vi "单参数加标流程.vi"(10 "流程类型":T1(ring), 11 "Slave ID":T3=enum."氨氮") -> ()   [LabVIEW 2016, in "质控单元V4.lvlib"]
panel:
  out "加标回收启动时间":timestamp
  out "水样测试启动时间":timestamp
  out "Next State":string
  in  "仪器加标回收启动计数":u16
  in  "仪器水样测试启动计数":u16
  in  "加标模块排液启动计数":u16
  in  "加标模块加标启动计数":u16
  in  "加标模块进样启动计数":u16
  in  "加标模块润洗启动计数":u16
  in  "采配水启动次数计数":u16
  in  "加标回收测试时间":timestamp
  in  "水样测试时间":timestamp
  in  "质控数据":T2
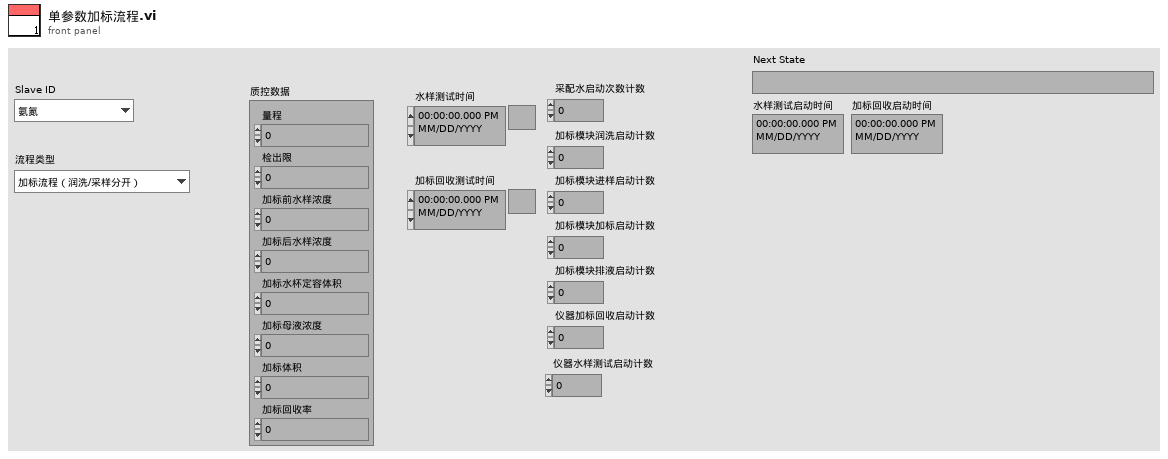
[diagram p1: front panel]
types:
  T1 = enum16{"加标流程（润洗/采样分开）", "加标流程（润洗/采样合并）", "加标流程（不启动采配水）", "水样测试（润洗/采样分开）", "水样测试（润洗/采样合并）", "水样测试（不启动采配水）"}
  T2 = cluster{"量程":dbl, "检出限":dbl, "加标前水样浓度":dbl, "加标后水样浓度":dbl, "加标水杯定容体积":dbl, "加标母液浓度":dbl, "加标体积":dbl, "加标回收率":dbl}
  T3 = typedef "质控单元V4.lvlib/质控slave id.ctl" = enum16{"null", "氨氮", "总磷", "总氮", "CODMn", "CODCr", "氨氮总磷", "总磷总氮"}
  T4 = cluster{"氨氮":bool, "总磷":bool, "总氮":bool, "CODMn":bool, "CODCr":bool, "氨氮总磷":bool, "总磷总氮":bool}
  T5 = cluster{"时间":timestamp, "参数":string, "数据类型":string, "加标前水样测试时间":timestamp, "加标前水样浓度值":sgl, "加标后水样浓度值":sgl, "加标母液浓度值":sgl, "加标体积":sgl, "加标水杯定容体积":sgl, "加标回收率":sgl}
  T6 = enum16{"待机", "润洗", "采样", "沉淀", "配水", "反冲洗", "储水", "结束"}
  T7 = typedef "质控单元V4.lvlib/质控流程控制.ctl" = enum16{"待机", "启动进样流程", "启动加标流程", "启动排液流程", "启动润洗流程", "停止流程"}
  T8 = enum16{"待机", "润洗", "进样", "定量", "加标", "等待取样", "排液", "异常停机"}
  T9 = enum16{"空闲", "水样测试", "标样核查", "零点核查", "跨度核查", "空白测试", "平行样测试", "加标回收", "空白校准", "标样校准", "初始化（清洗）"}
  T10 = cluster{"水样数据时间":timestamp, "水样实测值":sgl, "水样数据标识":string}
  T11 = cluster{"加标回收数据时间":timestamp, "加标回收实测值":sgl, "加标回收数据标识":string}
  T12 = typedef "质控单元V4.lvlib/质控仪器状态.ctl" = cluster{"运行状态":enum16{"待机", "润洗", "进样", "定量", "加标", "等待取样", "排液", "异常停机"}, "液位状态":enum16{"无感应", "有感应"}, "告警状态":enum16{"无告警", "液位故障告警", "注射泵异常"}, "当前步骤数":u16, "当前步骤剩余时间":u16, "当前步骤具体操作":enum16{"加标", "进样", "排液", "搅拌", "定量"}, "当前流程":enum16{"待机", "进样流程", "加标流程", "排液流程", "润洗流程"}}
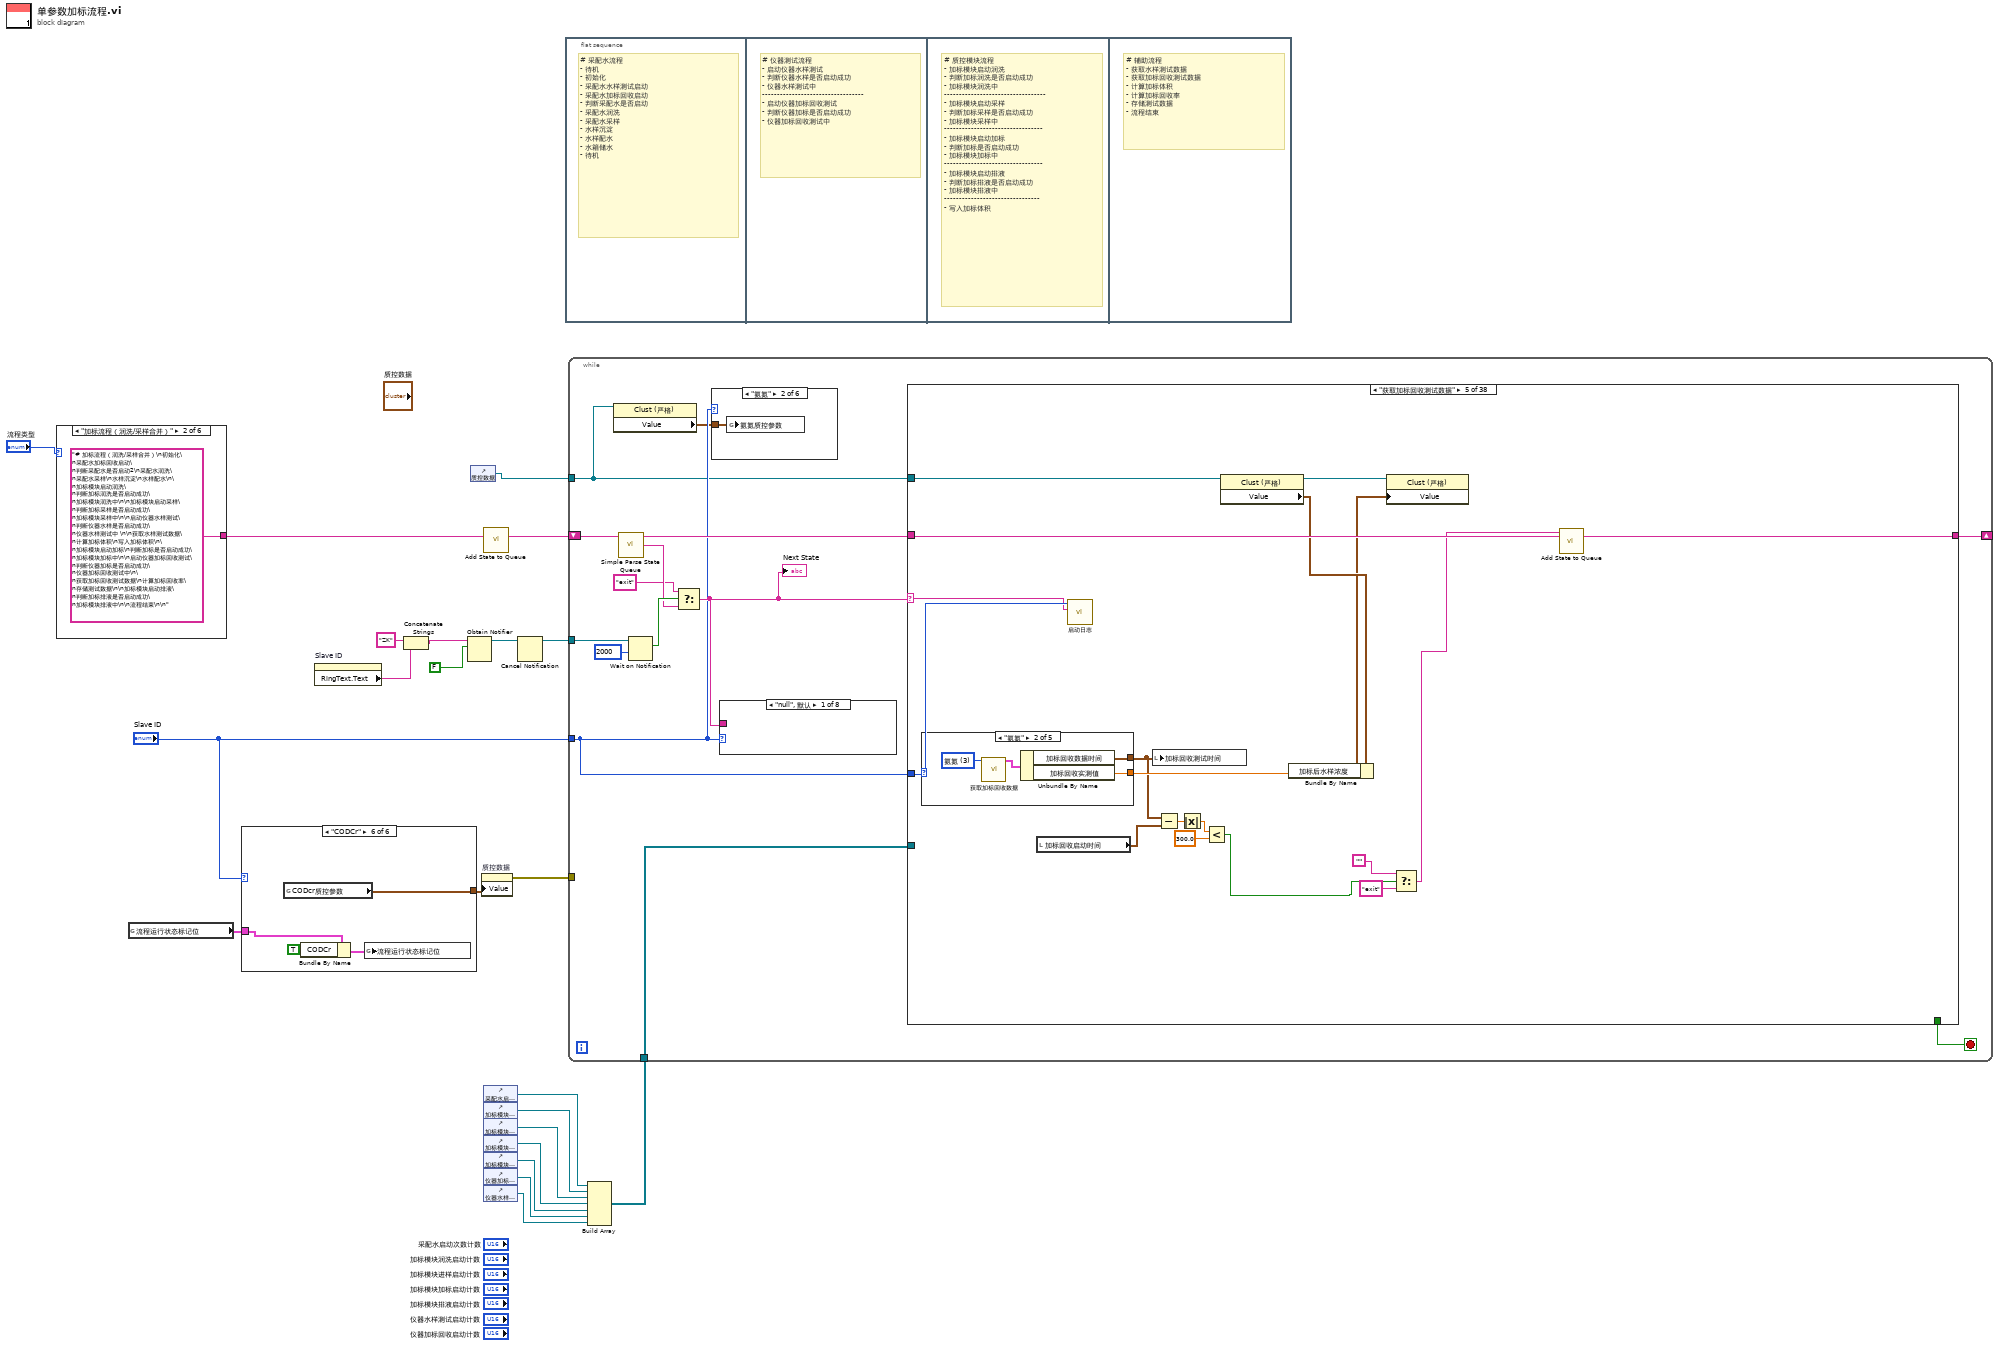
[diagram p0: block diagram]
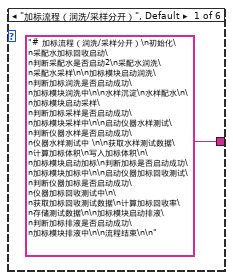
[diagram p2: hidden frame]
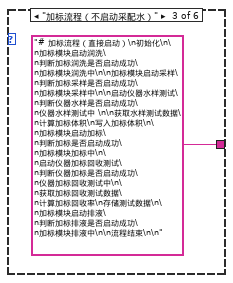
[diagram p3: hidden frame]
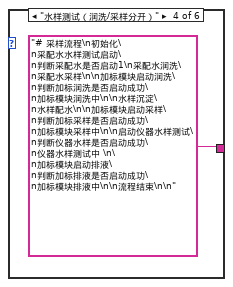
[diagram p4: hidden frame]
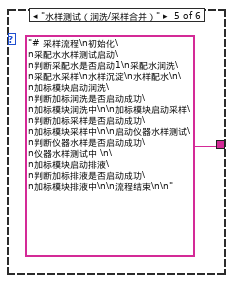
[diagram p5: hidden frame]
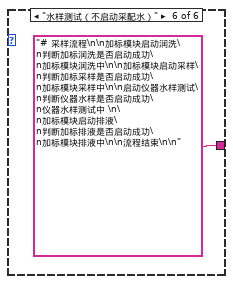
[diagram p6: hidden frame]
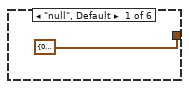
[diagram p7: hidden frame]
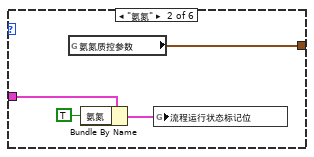
[diagram p8: hidden frame]
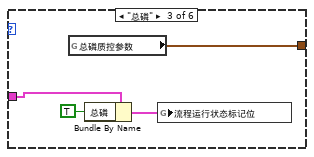
[diagram p9: hidden frame]
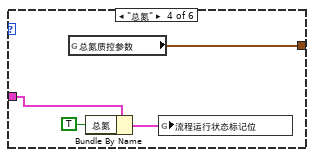
[diagram p10: hidden frame]
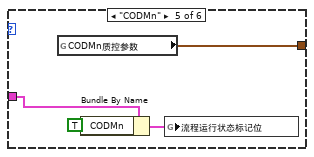
[diagram p11: hidden frame]
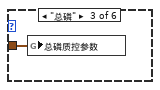
[diagram p13: hidden frame]
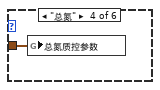
[diagram p14: hidden frame]
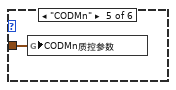
[diagram p15: hidden frame]
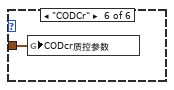
[diagram p16: hidden frame]
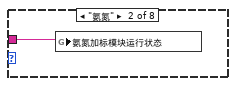
[diagram p17: hidden frame]
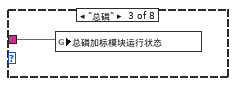
[diagram p18: hidden frame]
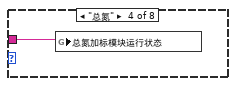
[diagram p19: hidden frame]
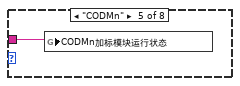
[diagram p20: hidden frame]
diagram:
  n1 = case shown="\"加标流程（润洗/采样合并）\"" "流程类型" {
    tunnel: ["# 加标流程（润洗/采样分开）\n初始化\n采配水加标回收启动\n判断采配水是否启动2\n采配水润洗\n采配水采样\n\n加标模块启动润洗\n判断加标润洗是否启动成功\n加标模块润洗中\n\n水样沉淀\n水样配水\n\n加标模块启动采样\n判断加标采样是否启动成功\n加标模块采样中\n\n启动仪器水样测试\n判断仪器水样是否启动成功\n仪器水样测试中 \n\n获取水样测试数据\n计算加标体积\n写入加标体积\n\n加标模块启动加标\n判断加标是否启动成功\n加标模块加标中\n\n启动仪器加标回收测试\n判断仪器加标是否启动成功\n仪器加标回收测试中\n\n获取加标回收测试数据\n计算加标回收率\n存储测试数据\n\n加标模块启动排液\n判断加标排液是否启动成功\n加标模块排液中\n\n流程结束\n\n" ("State(s) In (\"\")") "# 加标流程（润洗/采样合并）\n初始化\n采配水加标回收启动\n判断采配水是否启动2\n采配水润洗\n采配水采样\n水样沉淀\n水样配水\n\n加标模块启动润洗\n判断加标润洗是否启动成功\n加标模块润洗中\n\n加标模块启动采样\n判断加标采样是否启动成功\n加标模块采样中\n\n启动仪器水样测试\n判断仪器水样是否启动成功\n仪器水样测试中 \n\n获取水样测试数据\n计算加标体积\n写入加标体积\n\n加标模块启动加标\n判断加标是否启动成功\n加标模块加标中\n\n启动仪器加标回收测试\n判断仪器加标是否启动成功\n仪器加标回收测试中\n\n获取加标回收测试数据\n计算加标回收率\n存储测试数据\n\n加标模块启动排液\n判断加标排液是否启动成功\n加标模块排液中\n\n流程结束\n\n" ("State(s) In (\"\")") "# 加标流程（直接启动）\n初始化\n\n加标模块启动润洗\n判断加标润洗是否启动成功\n加标模块润洗中\n\n加标模块启动采样\n判断加标采样是否启动成功\n加标模块采样中\n\n启动仪器水样测试\n判断仪器水样是否启动成功\n仪器水样测试中 \n\n获取水样测试数据\n计算加标体积\n写入加标体积\n\n加标模块启动加标\n判断加标是否启动成功\n加标模块加标中\n\n启动仪器加标回收测试\n判断仪器加标是否启动成功\n仪器加标回收测试中\n\n获取加标回收测试数据\n计算加标回收率\n存储测试数据\n\n加标模块启动排液\n判断加标排液是否启动成功\n加标模块排液中\n\n流程结束\n\n" ("State(s) In (\"\")") "# 采样流程\n初始化\n采配水水样测试启动\n判断采配水是否启动1\n采配水润洗\n采配水采样\n\n加标模块启动润洗\n判断加标润洗是否启动成功\n加标模块润洗中\n\n水样沉淀\n水样配水\n\n加标模块启动采样\n判断加标采样是否启动成功\n加标模块采样中\n\n启动仪器水样测试\n判断仪器水样是否启动成功\n仪器水样测试中 \n\n加标模块启动排液\n判断加标排液是否启动成功\n加标模块排液中\n\n流程结束\n\n" ("State(s) In (\"\")") "# 采样流程\n初始化\n采配水水样测试启动\n判断采配水是否启动1\n采配水润洗\n采配水采样\n水样沉淀\n水样配水\n\n加标模块启动润洗\n判断加标润洗是否启动成功\n加标模块润洗中\n\n加标模块启动采样\n判断加标采样是否启动成功\n加标模块采样中\n\n启动仪器水样测试\n判断仪器水样是否启动成功\n仪器水样测试中 \n\n加标模块启动排液\n判断加标排液是否启动成功\n加标模块排液中\n\n流程结束\n\n" ("State(s) In (\"\")") "# 采样流程\n\n加标模块启动润洗\n判断加标润洗是否启动成功\n加标模块润洗中\n\n加标模块启动采样\n判断加标采样是否启动成功\n加标模块采样中\n\n启动仪器水样测试\n判断仪器水样是否启动成功\n仪器水样测试中 \n\n加标模块启动排液\n判断加标排液是否启动成功\n加标模块排液中\n\n流程结束\n\n" ("State(s) In (\"\")")] -> w2
    frame "加标流程（润洗/采样分开）", Default {
    }
    frame "加标流程（润洗/采样合并）" {
    }
    frame "加标流程（不启动采配水）" {
    }
    frame "水样测试（润洗/采样分开）" {
    }
    frame "水样测试（润洗/采样合并）" {
    }
    frame "水样测试（不启动采配水）" {
    }
  }
  n2 = global read "ZK非断电保存全局变量.vi" "流程运行状态标记位"() -> (w1:T4)
  n3 = case shown="\"CODCr\"" "Slave ID" {
    tunnel: [T2 {"量程"=0.0, "检出限"=0.0, "加标前水样浓度"=0.0, "加标后水样浓度"=0.0, "加标水杯定容体积"=0.0, "加标母液浓度"=0.0, "加标体积"=0.0, "加标回收率"=0.0} ("CODcr质控参数") w33 w37 w41 w45 w49] -> w13
    tunnel: w1 -> [_ w32 w34 w38 w42 w46]
    frame "null", Default {
    }
    frame "氨氮" {
      n4 = global read "ZK断电保存全局变量.vi" "氨氮质控参数"() -> (w33:T2)
      n5 = Bundle By Name(cluster=w32, "氨氮"=TRUE) -> (w31:T4)
      n6 = global write "ZK非断电保存全局变量.vi" "流程运行状态标记位"(w31) -> ()
    }
    frame "总磷" {
      n7 = global read "ZK断电保存全局变量.vi" "总磷质控参数"() -> (w37:T2)
      n8 = Bundle By Name(cluster=w34, "总磷"=TRUE ("氨氮")) -> (w36:T4)
      n9 = global write "ZK非断电保存全局变量.vi" "流程运行状态标记位"(w36) -> ()
    }
    frame "总氮" {
      n10 = global read "ZK断电保存全局变量.vi" "总氮质控参数"() -> (w41:T2)
      n11 = Bundle By Name(cluster=w38, "总氮"=TRUE ("氨氮")) -> (w40:T4)
      n12 = global write "ZK非断电保存全局变量.vi" "流程运行状态标记位"(w40) -> ()
    }
    frame "CODMn" {
      n13 = global read "ZK断电保存全局变量.vi" "CODMn质控参数"() -> (w45:T2)
      n14 = Bundle By Name(cluster=w42, "CODMn"=TRUE ("氨氮")) -> (w44:T4)
      n15 = global write "ZK非断电保存全局变量.vi" "流程运行状态标记位"(w44) -> ()
    }
    frame "CODCr" {
      n16 = global read "ZK断电保存全局变量.vi" "CODcr质控参数"() -> (w49:T2)
      n17 = Bundle By Name(cluster=w46, "CODCr"=TRUE ("氨氮")) -> (w48:T4)
      n18 = global write "ZK非断电保存全局变量.vi" "流程运行状态标记位"(w48) -> ()
    }
  }
  n19 = property on="Slave ID" class="Enum (严格)"() -> ("RingText.Text"=w22:string)  [unwired: 2 in, 2 out]
  n20 = Concatenate Strings("ZK" ("字符串"), w22) -> (w20:string)
  n21 = Obtain Notifier(name (unnamed)=w20, notification data type=FALSE) -> (notifier out=w18:refnum<notifier>)  [unwired: 2 in, 2 out]
  n22 = control-ref of="质控数据"() -> (w12:refnum<vi>)
  n23 = property on="质控数据" class="Clust (严格)"("Value"=w13) -> (error out=w15:errorcluster)  [unwired: 2 in, 1 out]
  n24 = call "Add State to Queue.vi"("State(s) In (\"\")"=w2) -> ("States Out"=w16:string)  [unwired: 14 in]
  n25 = control-ref of="采配水启动次数计数"() -> (w11:refnum<vi>)
  n26 = control-ref of="加标模块润洗启动计数"() -> (w10:refnum<vi>)
  n27 = control-ref of="加标模块进样启动计数"() -> (w9:refnum<vi>)
  n28 = control-ref of="加标模块加标启动计数"() -> (w8:refnum<vi>)
  n29 = control-ref of="加标模块排液启动计数"() -> (w7:refnum<vi>)
  n30 = control-ref of="仪器加标回收启动计数"() -> (w6:refnum<vi>)
  n31 = control-ref of="仪器水样测试启动计数"() -> (w5:refnum<vi>)
  n32 = Cancel Notification(0:w18) -> (8:w17:refnum<notifier>)  [unwired: 1 in, 2 out]
  n33 = flat-sequence {
    frame #0 {
      # "# 采配水流程\n- 待机\n- 初始化\n- 采配水水样测试启动\n- 采配水加标回收启动\n- 判断采配水是否启动\n- 采配水润洗\n- 采配水采样\n- 水样沉淀\n- 水样配水\n- 水箱储水\n- 待机"
    }
    frame #1 {
      # "# 仪器测试流程\n- 启动仪器水样测试\n- 判断仪器水样是否启动成功\n- 仪器水样测试中\n----------------------------------\n- 启动仪器加标回收测试\n- 判断仪器加标是否启动成功\n- 仪器加标回收测试中"
    }
    frame #2 {
      # "# 质控模块流程\n- 加标模块启动润洗\n- 判断加标润洗是否启动成功\n- 加标模块润洗中\n----------------------------------\n- 加标模块启动采样\n- 判断加标采样是否启动成功\n- 加标模块采样中\n---------------------------------\n- 加标模块启动加标\n- 判断加标是否启动成功\n- 加标模块加标中\n---------------------------------\n- 加标模块启动排液\n- 判断加标排液是否启动成功\n- 加标模块排液中\n--------------------------------\n- 写入加标体积"
    }
    frame #3 {
      # "# 辅助流程\n- 获取水样测试数据\n- 获取加标回收测试数据\n- 计算加标体积\n- 计算加标回收率\n- 存储测试数据\n- 流程结束"
    }
  }
  n34 = Build Array(w11, w10, w9, w8, w7, w6, w5) -> (w4:refnum<vi>[])
  n35 = while {
    tunnel: w17 -> [w62]
    tunnel: "Slave ID" -> [w53]
    shift-right: [w56] -> _
    shift-left: w16 -> [w63]
    tunnel: w15 -> [_]
    tunnel: w12 -> [w52]
    tunnel: w4 -> [w50]
    stop <- w55 stop-if-true
    n36 = property class="Clust (严格)"(reference=w52) -> ("Value"=w51:T2)  [unwired: 1 in, 2 out]
    n37 = call "Simple Parse State Queue.vi"("State Queue"=w63) -> ("Remain States"=w57:string, "Next State"=w59:string)  [unwired: 13 in]
    n38 = Wait on Notification(notifier=w62, timeout in ms (-1)=2000 ("超时毫秒(-1)")) -> (notification=w60:bool)  [unwired: 2 in, 3 out]
    n39 = Select(t="exit" ("State(s) In (\"\")"), s=w60, f=w59) -> (s? t:f=w54:string)
    "Next State" <- w54
    n40 = case shown="\"氨氮\"" w53 {
      tunnel: w51 -> [_ w64 w65 w66 w67 w68]
      frame "null", Default {
      }
      frame "氨氮" {
        n41 = global write "ZK断电保存全局变量.vi" "氨氮质控参数"(w64) -> ()
      }
      frame "总磷" {
        n42 = global write "ZK断电保存全局变量.vi" "总磷质控参数"(w65) -> ()
      }
      frame "总氮" {
        n43 = global write "ZK断电保存全局变量.vi" "总氮质控参数"(w66) -> ()
      }
      frame "CODMn" {
        n44 = global write "ZK断电保存全局变量.vi" "CODMn质控参数"(w67) -> ()
      }
      frame "CODCr" {
        n45 = global write "ZK断电保存全局变量.vi" "CODcr质控参数"(w68) -> ()
      }
    }
    n46 = case shown="\"null\", 默认" w53 {
      tunnel: w54 -> [_ w69 w70 w71 w72 w73 w74 w75]
      frame "null", Default {
      }
      frame "氨氮" {
        n47 = global write "ZK非断电保存全局变量.vi" "氨氮加标模块运行状态"(w69) -> ()
      }
      frame "总磷" {
        n48 = global write "ZK非断电保存全局变量.vi" "总磷加标模块运行状态"(w70) -> ()
      }
      frame "总氮" {
        n49 = global write "ZK非断电保存全局变量.vi" "总氮加标模块运行状态"(w71) -> ()
      }
      frame "CODMn" {
        n50 = global write "ZK非断电保存全局变量.vi" "CODMn加标模块运行状态"(w72) -> ()
      }
      frame "CODCr" {
        n51 = global write "ZK非断电保存全局变量.vi" "CODcr加标模块运行状态"(w73) -> ()
      }
      frame "氨氮总磷" {
        n52 = global write "ZK非断电保存全局变量.vi" "氨氮总磷加标模块运行状态"(w74) -> ()
      }
      frame "总磷总氮" {
        n53 = global write "ZK非断电保存全局变量.vi" "总磷总氮加标模块运行状态"(w75) -> ()
      }
    }
    n54 = case shown="\"获取加标回收测试数据\"" w54 {
      selector: w54 -> [_ _ w82 w103 w139 w167 w176 w184 w209 _ w240 w250 w260 w278 w297 w315 w332 w351 w365 _ w382 w393 w404 w414 w425 w436 w469 w502 w535 w569 w600 _ w633 w648 w664 w693 w720 w750]
      tunnel: w57 -> [w77 w79 w93 w111 w147 w175 w183 w200 w215 w239 w249 w259 w277 w279 w311 w326 w343 w362 w377 w381 w392 w403 w412 w424 w435 w453 w486 w519 w552 w581 w612 w631 w642 w657 w666 w710 w737 w756]
      tunnel: [w76 w78 w92 w110 w146 w174 w182 w199 w214 w238 w248 w258 w276 w295 w310 w325 w342 w361 w376 w380 w391 w402 w411 w423 w434 w452 w485 w518 w551 w580 w611 w630 w641 w656 w665 w709 w736 w755] -> w56
      tunnel: [_ _ _ _ _ _ _ _ TRUE _ _ _ _ _ _ _ _ _ _ _ _ _ _ _ _ _ _ _ _ _ _ _ _ _ _ _ _ _] -> w55
      tunnel: w53 -> [_ _ w83 w104 w140 w166 w177 w185 w210 _ w241 w251 w261 w280 w298 w316 w333 w352 w367 _ w383 w394 w407 w415 w426 w437 w470 w503 w536 w570 w601 _ w634 w649 w662 w694 w721 w748]
      tunnel: w52 -> [_ _ w88 w109 w145 w173 w181 w198 _ _ _ _ _ _ _ _ _ _ _ _ _ _ w410 _ _ _ _ _ _ _ _ _ _ _ _ _ _ _]
      tunnel: w50 -> [_ _ _ _ _ _ _ _ _ _ w247 w257 w265 w284 _ _ _ _ _ _ w385 w396 _ w418 w429 w441 w474 w507 w540 _ _ _ w637 w652 _ w698 w726 _]
      frame Default {
        n55 = call "Add State to Queue.vi"("State(s) In (\"\")"=w77) -> ("States Out"=w76:string)  [unwired: 14 in]
      }
      frame "-------------------# 辅助流程 #-------------------" {
        n56 = call "Add State to Queue.vi"("State(s) In (\"\")"=w79) -> ("States Out"=w78:string)  [unwired: 14 in]
      }
      frame "初始化" {
        w84 = 0.0 ("加标前水样浓度")
        w89 = u16 0 ("采配水启动次数计数")
        n57 = property class="Clust (严格)"(reference=w88) -> (reference out=w87:refnum<vi>, "Value"=w86:T2)  [unwired: 1 in, 1 out]
        n58 = call "ZK报警清除.vi"("Slave ID"=w83) -> ()  [unwired: 10 in, 1 out]
        n59 = Bundle By Name(cluster=w86, "加标前水样浓度"=w84, "加标后水样浓度"=w84, "加标体积"=w84, "加标回收率"=w84) -> (w85:T2)
        n60 = Concatenate Strings("----->>" ("字符串"), w82) -> (w81:string)
        n61 = call "启动日志.vi"("日志信息"=w81, "Slave ID"=w83) -> ()  [unwired: 9 in, 1 out]
        n62 = property class="Clust (严格)"(reference=w87, "Value"=w85) -> ()  [unwired: 1 in, 2 out]
        n63 = local write "水样测试时间"(timestamp(0 s since 1904-01-01) ("水样测试时间")) -> ()
        n64 = local write "加标回收测试时间"(timestamp(0 s since 1904-01-01) ("加标回收测试时间")) -> ()
        n65 = local write "采配水启动次数计数"(w89) -> ()
        n66 = local write "加标模块润洗启动计数"(w89) -> ()
        n67 = local write "加标模块进样启动计数"(w89) -> ()
        n68 = local write "加标模块加标启动计数"(w89) -> ()
        n69 = local write "加标模块排液启动计数"(w89) -> ()
        n70 = local write "仪器加标回收启动计数"(w89) -> ()
        n71 = local write "仪器水样测试启动计数"(w89) -> ()
        n72 = call "Add State to Queue.vi"("State(s) In (\"\")"=w93) -> ("States Out"=w92:string)  [unwired: 14 in]
      }
      frame "获取水样测试数据" {
        n73 = case shown="\"CODMn\"" w104 {
          tunnel: [sgl 0.0 ("水样实测值") w117 w121 w125 w129] -> w105
          tunnel: [timestamp(0 s since 1904-01-01) ("水样数据时间") w116 w120 w124 w128] -> w101
          frame "null", Default {
          }
          frame "氨氮" {
            w114 = u16 3 items=["总磷"=1, "总氮"=2, "氨氮"=3, "CODMn"=21] ("站号")
            n74 = call "获取水样测试数据.vi"("站号"=w114) -> ("测量数据区"=w115:T10)  [unwired: 10 in]
            n75 = Unbundle By Name(w115) -> ("水样数据时间"=w116:timestamp, "水样实测值"=w117:sgl)
          }
          frame "总磷" {
            w118 = u16 1 items=["总磷"=1, "总氮"=2, "氨氮"=3, "CODMn"=21] ("站号")
            n76 = call "获取水样测试数据.vi"("站号"=w118) -> ("测量数据区"=w119:T10)  [unwired: 10 in]
            n77 = Unbundle By Name(w119) -> ("水样数据时间"=w120:timestamp, "水样实测值"=w121:sgl)
          }
          frame "总氮" {
            w122 = u16 2 items=["总磷"=1, "总氮"=2, "氨氮"=3, "CODMn"=21] ("站号")
            n78 = call "获取水样测试数据.vi"("站号"=w122) -> ("测量数据区"=w123:T10)  [unwired: 10 in]
            n79 = Unbundle By Name(w123) -> ("水样数据时间"=w124:timestamp, "水样实测值"=w125:sgl)
          }
          frame "CODMn" {
            w126 = u16 21 items=["总磷"=1, "总氮"=2, "氨氮"=3, "CODMn"=21] ("站号")
            n80 = call "获取水样测试数据.vi"("站号"=w126) -> ("测量数据区"=w127:T10)  [unwired: 10 in]
            n81 = Unbundle By Name(w127) -> ("水样数据时间"=w128:timestamp, "水样实测值"=w129:sgl)
          }
        }
        n82 = call "启动日志.vi"("日志信息"=w103, "Slave ID"=w104) -> ()  [unwired: 9 in, 1 out]
        n83 = local read "水样测试启动时间"() -> (w102:timestamp)
        n84 = Subtract(x=w101, y=w102) -> (x-y=w100:dbl)
        n85 = local write "水样测试时间"(w101) -> ()
        n86 = Absolute Value(x=w100) -> (abs(x)=w99:dbl)
        n87 = property class="Clust (严格)"(reference=w109) -> (reference out=w108:refnum<vi>, "Value"=w107:T2)  [unwired: 1 in, 1 out]
        n88 = Less?(x=w99, y=300.0) -> (x < y?=w97:bool)
        n89 = Bundle By Name(cluster=w107, "加标前水样浓度"=w105) -> (w106:T2)
        n90 = property class="Clust (严格)"(reference=w108, "Value"=w106) -> ()  [unwired: 1 in, 2 out]
        n91 = Select(t="", s=w97, f="exit") -> (s? t:f=w95:string)
        n92 = call "Add State to Queue.vi"("State(s) In Front (\"\")"=w95, "State(s) In (\"\")"=w111) -> ("States Out"=w110:string)  [unwired: 13 in]
      }
      frame "获取加标回收测试数据" {
        n93 = case shown="\"氨氮\"" w140 {
          tunnel: [sgl 0.0 ("水样实测值") w153 w157 w161 w165] -> w141
          tunnel: [timestamp(0 s since 1904-01-01) ("加标回收数据时间") w152 w156 w160 w164] -> w135
          frame "null", Default {
          }
          frame "氨氮" {
            w150 = u16 3 items=["总磷"=1, "总氮"=2, "氨氮"=3, "CODMn"=21] ("站号")
            n94 = call "获取加标回收数据.vi"("站号"=w150) -> ("测量数据区"=w151:T11)  [unwired: 10 in]
            n95 = Unbundle By Name(w151) -> ("加标回收数据时间"=w152:timestamp, "加标回收实测值"=w153:sgl)
          }
          frame "总磷" {
            w154 = u16 1 items=["总磷"=1, "总氮"=2, "氨氮"=3, "CODMn"=21] ("站号")
            n96 = call "获取加标回收数据.vi"("站号"=w154) -> ("测量数据区"=w155:T11)  [unwired: 10 in]
            n97 = Unbundle By Name(w155) -> ("加标回收数据时间"=w156:timestamp, "加标回收实测值"=w157:sgl)
          }
          frame "总氮" {
            w158 = u16 2 items=["总磷"=1, "总氮"=2, "氨氮"=3, "CODMn"=21] ("站号")
            n98 = call "获取加标回收数据.vi"("站号"=w158) -> ("测量数据区"=w159:T11)  [unwired: 10 in]
            n99 = Unbundle By Name(w159) -> ("加标回收数据时间"=w160:timestamp, "加标回收实测值"=w161:sgl)
          }
          frame "CODMn" {
            w162 = u16 21 items=["总磷"=1, "总氮"=2, "氨氮"=3, "CODMn"=21] ("站号")
            n100 = call "获取加标回收数据.vi"("站号"=w162) -> ("测量数据区"=w163:T11)  [unwired: 10 in]
            n101 = Unbundle By Name(w163) -> ("加标回收数据时间"=w164:timestamp, "加标回收实测值"=w165:sgl)
          }
        }
        n102 = local read "加标回收启动时间"() -> (w136:timestamp)
        n103 = call "启动日志.vi"("日志信息"=w139, "Slave ID"=w140) -> ()  [unwired: 9 in, 1 out]
        n104 = local write "加标回收测试时间"(w135) -> ()
        n105 = Subtract(x=w135, y=w136) -> (x-y=w134:dbl)
        n106 = Absolute Value(x=w134) -> (abs(x)=w130:dbl)
        n107 = Less?(x=w130, y=300.0) -> (x < y?=w132:bool)
        n108 = property class="Clust (严格)"(reference=w145) -> (reference out=w144:refnum<vi>, "Value"=w143:T2)  [unwired: 1 in, 1 out]
        n109 = Bundle By Name(cluster=w143, "加标后水样浓度"=w141) -> (w142:T2)
        n110 = property class="Clust (严格)"(reference=w144, "Value"=w142) -> ()  [unwired: 1 in, 2 out]
        n111 = Select(t="", s=w132, f="exit") -> (s? t:f=w131:string)
        n112 = call "Add State to Queue.vi"("State(s) In Front (\"\")"=w131, "State(s) In (\"\")"=w147) -> ("States Out"=w146:string)  [unwired: 13 in]
      }
      frame "计算加标体积" {
        n113 = call "启动日志.vi"("日志信息"=w167, "Slave ID"=w166) -> ()  [unwired: 9 in, 1 out]
        n114 = property class="Clust (严格)"(reference=w173) -> (reference out=w172:refnum<vi>, "Value"=w171:T2)  [unwired: 1 in, 1 out]
        n115 = call "加标回收率计算.vi"("参数"=w171) -> ("参数 out"=w170:T2)  [unwired: 9 in, 1 out]
        n116 = Bundle By Name(cluster=w170, "加标回收率"=0.0) -> (w169:T2)
        n117 = property class="Clust (严格)"(reference=w172, "Value"=w169) -> ()  [unwired: 1 in, 2 out]
        n118 = call "Add State to Queue.vi"("State(s) In (\"\")"=w175) -> ("States Out"=w174:string)  [unwired: 14 in]
      }
      frame "计算加标回收率" {
        n119 = call "启动日志.vi"("日志信息"=w176, "Slave ID"=w177) -> ()  [unwired: 9 in, 1 out]
        n120 = property class="Clust (严格)"(reference=w181) -> (reference out=w180:refnum<vi>, "Value"=w179:T2)  [unwired: 1 in, 1 out]
        n121 = call "加标回收率计算.vi"("参数"=w179) -> ("参数 out"=w178:T2)  [unwired: 9 in, 1 out]
        n122 = property class="Clust (严格)"(reference=w180, "Value"=w178) -> ()  [unwired: 1 in, 2 out]
        n123 = call "Add State to Queue.vi"("State(s) In (\"\")"=w183) -> ("States Out"=w182:string)  [unwired: 14 in]
      }
      frame "存储测试数据" {
        n124 = case shown="\"总氮\"" w185 {
          tunnel: ["" "氨氮加标回收率" "总磷加标回收率" "总氮加标回收率" "CODMn加标回收率" "CODCr加标回收率"] -> w186
          frame "null", Default {
          }
          frame "氨氮" {
          }
          frame "总磷" {
          }
          frame "总氮" {
          }
          frame "CODMn" {
          }
          frame "CODCr" {
          }
        }
        n125 = property class="Clust (严格)"(reference=w198) -> ("Value"=w193:T2)  [unwired: 1 in, 2 out]
        n126 = Unbundle By Name(w193) -> ("加标前水样浓度"=w192:dbl, "加标后水样浓度"=w191:dbl, "加标母液浓度"=w190:dbl, "加标体积"=w189:dbl, "加标水杯定容体积"=w188:dbl, "加标回收率"=w187:dbl)
        n127 = call "启动日志.vi"("日志信息"=w184, "Slave ID"=w185) -> ()  [unwired: 9 in, 1 out]
        n128 = Bundle By Name(cluster=T5 {"时间"=timestamp(0 s since 1904-01-01), "参数"="", "数据类型"="N", "加标前水样测试时间"=timestamp(0 s since 1904-01-01), "加标前水样浓度值"=0.0, "加标后水样浓度值"=0.0, "加标母液浓度值"=0.0, "加标体积"=0.0, "加标水杯定容体积"=0.0, "加标回收率"=0.0} ("data in"), "时间"="加标回收测试时间", "参数"=w186, "加标前水样测试时间"="水样测试时间", "加标前水样浓度值"=w192, "加标后水样浓度值"=w191, "加标母液浓度值"=w190, "加标体积"=w189, "加标水杯定容体积"=w188, "加标回收率"=w187) -> (w196:T5)
        n129 = call "data insert.vi"("data in"=w196) -> ()  [unwired: 10 in, 1 out]
        n130 = call "Add State to Queue.vi"("State(s) In (\"\")"=w200) -> ("States Out"=w199:string)  [unwired: 14 in]
      }
      frame "流程结束" {
        n131 = Concatenate Strings("----->>" ("字符串"), w209) -> (w208:string)
        n132 = call "启动日志.vi"("日志信息"=w208, "Slave ID"=w210) -> ()  [unwired: 9 in, 1 out]
        n133 = global read "ZK非断电保存全局变量.vi" "流程运行状态标记位"() -> (w212:T4)
        n134 = case shown="\"总磷\"" w210 {
          tunnel: "空闲" -> [_ w216 w217 w218 w219 w220 w221 w222]
          frame "null", Default {
          }
          frame "氨氮" {
            n135 = global write "ZK非断电保存全局变量.vi" "氨氮加标模块运行状态"(w216) -> ()
          }
          frame "总磷" {
            n136 = global write "ZK非断电保存全局变量.vi" "总磷加标模块运行状态"(w217) -> ()
          }
          frame "总氮" {
            n137 = global write "ZK非断电保存全局变量.vi" "总氮加标模块运行状态"(w218) -> ()
          }
          frame "CODMn" {
            n138 = global write "ZK非断电保存全局变量.vi" "CODMn加标模块运行状态"(w219) -> ()
          }
          frame "CODCr" {
            n139 = global write "ZK非断电保存全局变量.vi" "CODcr加标模块运行状态"(w220) -> ()
          }
          frame "氨氮总磷" {
            n140 = global write "ZK非断电保存全局变量.vi" "氨氮总磷加标模块运行状态"(w221) -> ()
          }
          frame "总磷总氮" {
            n141 = global write "ZK非断电保存全局变量.vi" "总磷总氮加标模块运行状态"(w222) -> ()
          }
        }
        n142 = case shown="\"氨氮\"" w210 {
          tunnel: w212 -> [_ w225 w226 w229 w232 w235]
          frame "null", Default {
          }
          frame "氨氮" {
            n143 = Bundle By Name(cluster=w225, "氨氮"=FALSE) -> (w224:T4)
            n144 = global write "ZK非断电保存全局变量.vi" "流程运行状态标记位"(w224) -> ()
          }
          frame "总磷" {
            n145 = Bundle By Name(cluster=w226, "总磷"=FALSE ("氨氮")) -> (w228:T4)
            n146 = global write "ZK非断电保存全局变量.vi" "流程运行状态标记位"(w228) -> ()
          }
          frame "总氮" {
            n147 = Bundle By Name(cluster=w229, "总氮"=FALSE ("氨氮")) -> (w231:T4)
            n148 = global write "ZK非断电保存全局变量.vi" "流程运行状态标记位"(w231) -> ()
          }
          frame "CODMn" {
            n149 = Bundle By Name(cluster=w232, "CODMn"=FALSE ("氨氮")) -> (w234:T4)
            n150 = global write "ZK非断电保存全局变量.vi" "流程运行状态标记位"(w234) -> ()
          }
          frame "CODCr" {
            n151 = Bundle By Name(cluster=w235, "CODCr"=FALSE ("氨氮")) -> (w237:T4)
            n152 = global write "ZK非断电保存全局变量.vi" "流程运行状态标记位"(w237) -> ()
          }
        }
        n153 = call "Add State to Queue.vi"("State(s) In (\"\")"=w215) -> ("States Out"=w214:string)  [unwired: 14 in]
      }
      frame "-------------------# 采配水流程 #-------------------" {
        n154 = call "Add State to Queue.vi"("State(s) In (\"\")"=w239) -> ("States Out"=w238:string)  [unwired: 14 in]
      }
      frame "采配水水样测试启动" {
        n155 = Index Array(array=w247) -> (element=w246:refnum<vi>)  [unwired: 1 in]
        n156 = property class="DigNum (严格)"(reference=w246) -> (reference out=w245:refnum<vi>, "Value"=w244:u16)  [unwired: 1 in, 1 out]
        n157 = call "启动日志.vi"("日志信息"=w240, "Slave ID"=w241) -> ()  [unwired: 9 in, 1 out]
        n158 = Increment(x=w244) -> (x+1=w243:u16)
        n159 = property class="DigNum (严格)"(reference=w245, "Value"=w243) -> ()  [unwired: 1 in, 2 out]
        n160 = call "采配水启动器.vi"("启动/停止命令"=enum16{"待机", "水样测试", "停止", "加标回收"}."水样测试") -> ()  [unwired: 10 in, 1 out]
        n161 = call "Add State to Queue.vi"("State(s) In (\"\")"=w249) -> ("States Out"=w248:string)  [unwired: 14 in]
      }
      frame "采配水加标回收启动" {
        n162 = Index Array(array=w257) -> (element=w256:refnum<vi>)  [unwired: 1 in]
        n163 = property class="DigNum (严格)"(reference=w256) -> (reference out=w255:refnum<vi>, "Value"=w254:u16)  [unwired: 1 in, 1 out]
        n164 = call "启动日志.vi"("日志信息"=w250, "Slave ID"=w251) -> ()  [unwired: 9 in, 1 out]
        n165 = Increment(x=w254) -> (x+1=w253:u16)
        n166 = property class="DigNum (严格)"(reference=w255, "Value"=w253) -> ()  [unwired: 1 in, 2 out]
        n167 = call "采配水启动器.vi"("启动/停止命令"=enum16{"待机", "水样测试", "停止", "加标回收"}."加标回收") -> ()  [unwired: 10 in, 1 out]
        n168 = call "Add State to Queue.vi"("State(s) In (\"\")"=w259) -> ("States Out"=w258:string)  [unwired: 14 in]
      }
      frame "判断采配水是否启动1" {
        n169 = Index Array(array=w265, index=0 ("索引")) -> (element=w264:refnum<vi>)
        n170 = property class="DigNum (严格)"(reference=w264) -> ("Value"=w263:u16)  [unwired: 1 in, 2 out]
        n171 = call "获取采配水运行状态.vi"() -> ("运行流程"=w275:T6)  [unwired: 10 in, 1 out]
        n172 = call "启动日志.vi"("日志信息"=w260, "Slave ID"=w261) -> ()  [unwired: 9 in, 1 out]
        n173 = Equal?(x=T6."待机" ("运行流程"), y=w275) -> (x = y?=w274:bool)
        n174 = Select(t="采配水水样测试启动\n判断采配水是否启动1" ("State(s) In (\"\")"), s=w274, f="") -> (s? t:f=w268:string)
        n175 = Greater Or Equal?(x=w263, y=u16 5) -> (x >= y?=w270:bool)
        n176 = Select(t="流程结束" ("State(s) In (\"\")"), s=w270, f=w268) -> (s? t:f=w267:string)
        n177 = call "Add State to Queue.vi"("State(s) In Front (\"\")"=w267, "State(s) In (\"\")"=w277) -> ("States Out"=w276:string)  [unwired: 13 in]
      }
      frame "判断采配水是否启动2" {
        n178 = Index Array(array=w284, index=0 ("索引")) -> (element=w283:refnum<vi>)
        n179 = property class="DigNum (严格)"(reference=w283) -> ("Value"=w282:u16)  [unwired: 1 in, 2 out]
        n180 = call "获取采配水运行状态.vi"() -> ("运行流程"=w294:T6)  [unwired: 10 in, 1 out]
        n181 = call "启动日志.vi"("日志信息"=w278, "Slave ID"=w280) -> ()  [unwired: 9 in, 1 out]
        n182 = Equal?(x=T6."待机" ("运行流程"), y=w294) -> (x = y?=w293:bool)
        n183 = Select(t="采配水加标回收启动\n判断采配水是否启动2" ("State(s) In (\"\")"), s=w293, f="") -> (s? t:f=w287:string)
        n184 = Greater Or Equal?(x=w282, y=u16 5) -> (x >= y?=w289:bool)
        n185 = Select(t="流程结束" ("State(s) In (\"\")"), s=w289, f=w287) -> (s? t:f=w286:string)
        n186 = call "Add State to Queue.vi"("State(s) In Front (\"\")"=w286, "State(s) In (\"\")"=w279) -> ("States Out"=w295:string)  [unwired: 13 in]
      }
      frame "采配水润洗" {
        n187 = call "获取采配水运行状态.vi"() -> ("运行流程"=w305:T6)  [unwired: 10 in, 1 out]
        n188 = First Call?() -> (First Call?: T/F=w296:bool)
        n189 = case shown="真" w296 {
          tunnel: w298 -> [_ w313]
          tunnel: w297 -> [_ w312]
          frame False {
          }
          frame True {
            n190 = call "启动日志.vi"("日志信息"=w312, "Slave ID"=w313) -> ()  [unwired: 9 in, 1 out]
          }
        }
        n191 = Less?(x=w305, y=T6."采样" ("运行流程")) -> (x < y?=w308:bool)
        n192 = Greater?(x=w305, y=T6."待机" ("运行流程")) -> (0:w309:bool)
        n193 = And(x=w308, y=w309) -> (x .and. y?=w307:bool)
        n194 = Select(t=w297, s=w307, f="") -> (s? t:f=w302:string)
        n195 = Equal To 0?(x=w305) -> (x = 0?=w304:bool)
        n196 = Select(t="流程结束" ("State(s) In (\"\")"), s=w304, f=w302) -> (s? t:f=w301:string)
        n197 = call "Add State to Queue.vi"("State(s) In Front (\"\")"=w301, "State(s) In (\"\")"=w311) -> ("States Out"=w310:string)  [unwired: 13 in]
      }
      frame "采配水采样" {
        n198 = First Call?() -> (First Call?: T/F=w314:bool)
        n199 = call "获取采配水运行状态.vi"() -> ("运行流程"=w318:T6)  [unwired: 10 in, 1 out]
        n200 = case shown="真" w314 {
          tunnel: w316 -> [_ w328]
          tunnel: w315 -> [_ w327]
          frame False {
          }
          frame True {
            n201 = call "启动日志.vi"("日志信息"=w327, "Slave ID"=w328) -> ()  [unwired: 9 in, 1 out]
          }
        }
        n202 = Equal?(x=T6."采样" ("运行流程"), y=w318) -> (x = y?=w317:bool)
        n203 = Select(t=w315, s=w317, f="") -> (s? t:f=w321:string)
        n204 = Equal To 0?(x=w318) -> (x = 0?=w323:bool)
        n205 = Select(t="流程结束" ("State(s) In (\"\")"), s=w323, f=w321) -> (s? t:f=w320:string)
        n206 = call "Add State to Queue.vi"("State(s) In Front (\"\")"=w320, "State(s) In (\"\")"=w326) -> ("States Out"=w325:string)  [unwired: 13 in]
      }
      frame "水样沉淀" {
        n207 = First Call?() -> (First Call?: T/F=w331:bool)
        n208 = global read "系统交互.vi" "站点类型"() -> (w329:enum16{"一体站", "固定站"})
        n209 = case shown="\"一体站\", 默认" w329 {
          tunnel: [w345 _] -> w330
          frame "一体站", Default {
            n210 = First Call?() -> (First Call?: T/F=w344:bool)
            n211 = case shown="真" w344 {
              tunnel: [_ w346] -> w345
              frame False {
              }
              frame True {
                n212 = call "质控模块润洗OK命令.vi"("质控润洗OK"=TRUE) -> ("error out"=w346:errorcluster)  [unwired: 10 in]
              }
            }
          }
          frame "固定站" {
          }
        }
        n213 = case shown="真" w331 {
          tunnel: w333 -> [_ w349]
          tunnel: w332 -> [_ w348]
          frame False {
          }
          frame True {
            n214 = call "启动日志.vi"("日志信息"=w348, "Slave ID"=w349) -> ()  [unwired: 9 in, 1 out]
          }
        }
        n215 = call "获取采配水运行状态.vi"("error in (no error)"=w330) -> ("运行流程"=w339:T6)  [unwired: 9 in, 1 out]
        n216 = Equal?(x=T6."沉淀" ("运行流程"), y=w339) -> (x = y?=w341:bool)
        n217 = Equal To 0?(x=w339) -> (x = 0?=w338:bool)
        n218 = Select(t=w332, s=w341, f="") -> (s? t:f=w336:string)
        n219 = Select(t="流程结束" ("State(s) In (\"\")"), s=w338, f=w336) -> (s? t:f=w335:string)
        n220 = call "Add State to Queue.vi"("State(s) In Front (\"\")"=w335, "State(s) In (\"\")"=w343) -> ("States Out"=w342:string)  [unwired: 13 in]
      }
      frame "水样配水" {
        n221 = First Call?() -> (First Call?: T/F=w350:bool)
        n222 = call "获取采配水运行状态.vi"() -> ("运行流程"=w359:T6)  [unwired: 10 in, 1 out]
        n223 = case shown="真" w350 {
          tunnel: w352 -> [_ w364]
          tunnel: w351 -> [_ w363]
          frame False {
          }
          frame True {
            n224 = call "启动日志.vi"("日志信息"=w363, "Slave ID"=w364) -> ()  [unwired: 9 in, 1 out]
          }
        }
        n225 = Equal?(x=T6."配水" ("运行流程"), y=w359) -> (x = y?=w360:bool)
        n226 = Equal To 0?(x=w359) -> (x = 0?=w358:bool)
        n227 = Select(t="", s=w360, f=w351) -> (s? t:f=w356:string)
        n228 = Select(t="流程结束" ("State(s) In (\"\")"), s=w358, f=w356) -> (s? t:f=w355:string)
        n229 = call "Add State to Queue.vi"("State(s) In Front (\"\")"=w355, "State(s) In (\"\")"=w362) -> ("States Out"=w361:string)  [unwired: 13 in]
      }
      frame "水箱储水" {
        n230 = First Call?() -> (First Call?: T/F=w366:bool)
        n231 = case shown="真" w366 {
          tunnel: w367 -> [_ w379]
          tunnel: w365 -> [_ w378]
          frame False {
          }
          frame True {
            n232 = call "启动日志.vi"("日志信息"=w378, "Slave ID"=w379) -> ()  [unwired: 9 in, 1 out]
          }
        }
        n233 = call "获取采配水运行状态.vi"() -> ("运行流程"=w374:T6)  [unwired: 10 in, 1 out]
        n234 = Equal?(x=T6."储水" ("运行流程"), y=w374) -> (x = y?=w375:bool)
        n235 = Equal To 0?(x=w374) -> (x = 0?=w373:bool)
        n236 = Select(t="", s=w375, f=w365) -> (s? t:f=w371:string)
        n237 = Select(t="流程结束" ("State(s) In (\"\")"), s=w373, f=w371) -> (s? t:f=w370:string)
        n238 = call "Add State to Queue.vi"("State(s) In Front (\"\")"=w370, "State(s) In (\"\")"=w377) -> ("States Out"=w376:string)  [unwired: 13 in]
      }
      frame "-------------------# 质控模块流程 #-------------------" {
        n239 = call "Add State to Queue.vi"("State(s) In (\"\")"=w381) -> ("States Out"=w380:string)  [unwired: 14 in]
      }
      frame "加标模块启动润洗" {
        n240 = Index Array(array=w385, index=1 ("索引")) -> (element=w389:refnum<vi>)
        n241 = call "ZK流程控制.vi"("流程控制"=质控流程控制."启动润洗流程", "Slave ID"=w383) -> ()  [unwired: 9 in, 1 out]
        n242 = property class="DigNum (严格)"(reference=w389) -> (reference out=w388:refnum<vi>, "Value"=w387:u16)  [unwired: 1 in, 1 out]
        n243 = Increment(x=w387) -> (x+1=w386:u16)
        n244 = property class="DigNum (严格)"(reference=w388, "Value"=w386) -> ()  [unwired: 1 in, 2 out]
        n245 = call "启动日志.vi"("日志信息"=w382, "Slave ID"=w383) -> ()  [unwired: 9 in, 1 out]
        n246 = call "Add State to Queue.vi"("State(s) In (\"\")"=w392) -> ("States Out"=w391:string)  [unwired: 14 in]
      }
      frame "加标模块启动采样" {
        n247 = Index Array(array=w396, index=2 ("索引")) -> (element=w400:refnum<vi>)
        n248 = call "ZK流程控制.vi"("流程控制"=质控流程控制."启动进样流程", "Slave ID"=w394) -> ()  [unwired: 9 in, 1 out]
        n249 = property class="DigNum (严格)"(reference=w400) -> (reference out=w399:refnum<vi>, "Value"=w398:u16)  [unwired: 1 in, 1 out]
        n250 = Increment(x=w398) -> (x+1=w397:u16)
        n251 = property class="DigNum (严格)"(reference=w399, "Value"=w397) -> ()  [unwired: 1 in, 2 out]
        n252 = call "启动日志.vi"("日志信息"=w393, "Slave ID"=w394) -> ()  [unwired: 9 in, 1 out]
        n253 = call "Add State to Queue.vi"("State(s) In (\"\")"=w403) -> ("States Out"=w402:string)  [unwired: 14 in]
      }
      frame "写入加标体积" {
        n254 = property class="Clust (严格)"(reference=w410) -> ("Value"=w409:T2)  [unwired: 1 in, 2 out]
        n255 = Unbundle By Name(w409) -> ("加标体积"=w408:dbl)
        n256 = call "启动日志.vi"("日志信息"=w404, "Slave ID"=w407) -> ()  [unwired: 9 in, 1 out]
        n257 = call "ZK加标体积写入.vi"("加标体积"=w408, "Slave ID"=w407) -> ("error out"=w406:errorcluster)  [unwired: 9 in]
        n258 = case shown="无错误" w406 {
          tunnel: [_ w413] -> w405
          tunnel: w404 -> [_ w413]
          frame No Error {
          }
          frame Error {
          }
        }
        n259 = call "Add State to Queue.vi"("State(s) In Front (\"\")"=w405, "State(s) In (\"\")"=w412) -> ("States Out"=w411:string)  [unwired: 13 in]
      }
      frame "加标模块启动加标" {
        n260 = Index Array(array=w418, index=3 ("索引")) -> (element=w417:refnum<vi>)
        n261 = call "ZK流程控制.vi"("流程控制"=质控流程控制."启动加标流程", "Slave ID"=w415) -> ()  [unwired: 9 in, 1 out]
        n262 = property class="DigNum (严格)"(reference=w417) -> (reference out=w421:refnum<vi>, "Value"=w420:u16)  [unwired: 1 in, 1 out]
        n263 = call "启动日志.vi"("日志信息"=w414, "Slave ID"=w415) -> ()  [unwired: 9 in, 1 out]
        n264 = Increment(x=w420) -> (x+1=w419:u16)
        n265 = property class="DigNum (严格)"(reference=w421, "Value"=w419) -> ()  [unwired: 1 in, 2 out]
        n266 = call "Add State to Queue.vi"("State(s) In (\"\")"=w424) -> ("States Out"=w423:string)  [unwired: 14 in]
      }
      frame "加标模块启动排液" {
        n267 = Index Array(array=w429, index=4 ("索引")) -> (element=w428:refnum<vi>)
        n268 = property class="DigNum (严格)"(reference=w428) -> (reference out=w432:refnum<vi>, "Value"=w431:u16)  [unwired: 1 in, 1 out]
        n269 = call "ZK流程控制.vi"("流程控制"=质控流程控制."启动排液流程", "Slave ID"=w426) -> ()  [unwired: 9 in, 1 out]
        n270 = call "启动日志.vi"("日志信息"=w425, "Slave ID"=w426) -> ()  [unwired: 9 in, 1 out]
        n271 = Increment(x=w431) -> (x+1=w430:u16)
        n272 = property class="DigNum (严格)"(reference=w432, "Value"=w430) -> ()  [unwired: 1 in, 2 out]
        n273 = call "Add State to Queue.vi"("State(s) In (\"\")"=w435) -> ("States Out"=w434:string)  [unwired: 14 in]
      }
      frame "判断加标润洗是否启动成功" {
        n274 = Index Array(array=w441, index=1 ("索引")) -> (element=w440:refnum<vi>)
        n275 = case shown="\"null\", 默认" w437 {
          tunnel: [T8."异常停机" ("运行状态") w455 w457 w459 w461 w463 w465 w467] -> w450
          frame "null", Default {
          }
          frame "氨氮" {
            n276 = global read "ZK非断电保存全局变量.vi" "氨氮质控仪器状态"() -> (w456:T12)
            n277 = Unbundle By Name(w456) -> ("运行状态"=w455:T8)
          }
          frame "总磷" {
            n278 = global read "ZK非断电保存全局变量.vi" "总磷质控仪器状态"() -> (w458:T12)
            n279 = Unbundle By Name(w458) -> ("运行状态"=w457:T8)
          }
          frame "总氮" {
            n280 = global read "ZK非断电保存全局变量.vi" "总氮质控仪器状态"() -> (w460:T12)
            n281 = Unbundle By Name(w460) -> ("运行状态"=w459:T8)
          }
          frame "CODMn" {
            n282 = global read "ZK非断电保存全局变量.vi" "CODMn质控仪器状态"() -> (w462:T12)
            n283 = Unbundle By Name(w462) -> ("运行状态"=w461:T8)
          }
          frame "CODCr" {
            n284 = global read "ZK非断电保存全局变量.vi" "CODCr质控仪器状态"() -> (w464:T12)
            n285 = Unbundle By Name(w464) -> ("运行状态"=w463:T8)
          }
          frame "氨氮总磷" {
            n286 = global read "ZK非断电保存全局变量.vi" "氨氮总磷质控仪器状态"() -> (w466:T12)
            n287 = Unbundle By Name(w466) -> ("运行状态"=w465:T8)
          }
          frame "总磷总氮" {
            n288 = global read "ZK非断电保存全局变量.vi" "总磷总氮质控仪器状态"() -> (w468:T12)
            n289 = Unbundle By Name(w468) -> ("运行状态"=w467:T8)
          }
        }
        n290 = property class="DigNum (严格)"(reference=w440) -> ("Value"=w439:u16)  [unwired: 1 in, 2 out]
        n291 = call "启动日志.vi"("日志信息"=w436, "Slave ID"=w437) -> ()  [unwired: 9 in, 1 out]
        n292 = Not Equal?(x=w450, y=T8."待机") -> (x != y?=w449:bool)
        n293 = Greater Or Equal?(x=w439, y=u16 5) -> (x >= y?=w442:bool)
        n294 = Select(t="", s=w449, f="加标模块启动润洗\n判断加标润洗是否启动成功" ("State(s) In (\"\")")) -> (s? t:f=w446:string)
        n295 = Select(t="流程结束" ("State(s) In (\"\")"), s=w442, f=w446) -> (s? t:f=w444:string)
        n296 = call "Add State to Queue.vi"("State(s) In Front (\"\")"=w444, "State(s) In (\"\")"=w453) -> ("States Out"=w452:string)  [unwired: 13 in]
      }
      frame "判断加标采样是否启动成功" {
        n297 = case shown="\"CODMn\"" w470 {
          tunnel: [T8."异常停机" ("运行状态") w488 w490 w492 w494 w496 w498 w500] -> w483
          frame "null", Default {
          }
          frame "氨氮" {
            n298 = global read "ZK非断电保存全局变量.vi" "氨氮质控仪器状态"() -> (w489:T12)
            n299 = Unbundle By Name(w489) -> ("运行状态"=w488:T8)
          }
          frame "总磷" {
            n300 = global read "ZK非断电保存全局变量.vi" "总磷质控仪器状态"() -> (w491:T12)
            n301 = Unbundle By Name(w491) -> ("运行状态"=w490:T8)
          }
          frame "总氮" {
            n302 = global read "ZK非断电保存全局变量.vi" "总氮质控仪器状态"() -> (w493:T12)
            n303 = Unbundle By Name(w493) -> ("运行状态"=w492:T8)
          }
          frame "CODMn" {
            n304 = global read "ZK非断电保存全局变量.vi" "CODMn质控仪器状态"() -> (w495:T12)
            n305 = Unbundle By Name(w495) -> ("运行状态"=w494:T8)
          }
          frame "CODCr" {
            n306 = global read "ZK非断电保存全局变量.vi" "CODCr质控仪器状态"() -> (w497:T12)
            n307 = Unbundle By Name(w497) -> ("运行状态"=w496:T8)
          }
          frame "氨氮总磷" {
            n308 = global read "ZK非断电保存全局变量.vi" "氨氮总磷质控仪器状态"() -> (w499:T12)
            n309 = Unbundle By Name(w499) -> ("运行状态"=w498:T8)
          }
          frame "总磷总氮" {
            n310 = global read "ZK非断电保存全局变量.vi" "总磷总氮质控仪器状态"() -> (w501:T12)
            n311 = Unbundle By Name(w501) -> ("运行状态"=w500:T8)
          }
        }
        n312 = Index Array(array=w474, index=2 ("索引")) -> (element=w473:refnum<vi>)
        n313 = property class="DigNum (严格)"(reference=w473) -> ("Value"=w472:u16)  [unwired: 1 in, 2 out]
        n314 = call "启动日志.vi"("日志信息"=w469, "Slave ID"=w470) -> ()  [unwired: 9 in, 1 out]
        n315 = Not Equal?(x=w483, y=T8."待机") -> (x != y?=w482:bool)
        n316 = Greater Or Equal?(x=w472, y=u16 5) -> (x >= y?=w475:bool)
        n317 = Select(t="", s=w482, f="加标模块启动采样\n判断加标采样是否启动成功" ("State(s) In (\"\")")) -> (s? t:f=w479:string)
        n318 = Select(t="流程结束" ("State(s) In (\"\")"), s=w475, f=w479) -> (s? t:f=w477:string)
        n319 = call "Add State to Queue.vi"("State(s) In Front (\"\")"=w477, "State(s) In (\"\")"=w486) -> ("States Out"=w485:string)  [unwired: 13 in]
      }
      frame "判断加标是否启动成功" {
        n320 = case shown="\"null\", 默认" w503 {
          tunnel: [T8."异常停机" ("运行状态") w521 w523 w525 w527 w529 w531 w533] -> w516
          frame "null", Default {
          }
          frame "氨氮" {
            n321 = global read "ZK非断电保存全局变量.vi" "氨氮质控仪器状态"() -> (w522:T12)
            n322 = Unbundle By Name(w522) -> ("运行状态"=w521:T8)
          }
          frame "总磷" {
            n323 = global read "ZK非断电保存全局变量.vi" "总磷质控仪器状态"() -> (w524:T12)
            n324 = Unbundle By Name(w524) -> ("运行状态"=w523:T8)
          }
          frame "总氮" {
            n325 = global read "ZK非断电保存全局变量.vi" "总氮质控仪器状态"() -> (w526:T12)
            n326 = Unbundle By Name(w526) -> ("运行状态"=w525:T8)
          }
          frame "CODMn" {
            n327 = global read "ZK非断电保存全局变量.vi" "CODMn质控仪器状态"() -> (w528:T12)
            n328 = Unbundle By Name(w528) -> ("运行状态"=w527:T8)
          }
          frame "CODCr" {
            n329 = global read "ZK非断电保存全局变量.vi" "CODCr质控仪器状态"() -> (w530:T12)
            n330 = Unbundle By Name(w530) -> ("运行状态"=w529:T8)
          }
          frame "氨氮总磷" {
            n331 = global read "ZK非断电保存全局变量.vi" "氨氮总磷质控仪器状态"() -> (w532:T12)
            n332 = Unbundle By Name(w532) -> ("运行状态"=w531:T8)
          }
          frame "总磷总氮" {
            n333 = global read "ZK非断电保存全局变量.vi" "总磷总氮质控仪器状态"() -> (w534:T12)
            n334 = Unbundle By Name(w534) -> ("运行状态"=w533:T8)
          }
        }
        n335 = Index Array(array=w507, index=3 ("索引")) -> (element=w506:refnum<vi>)
        n336 = property class="DigNum (严格)"(reference=w506) -> ("Value"=w505:u16)  [unwired: 1 in, 2 out]
        n337 = call "启动日志.vi"("日志信息"=w502, "Slave ID"=w503) -> ()  [unwired: 9 in, 1 out]
        n338 = Greater Or Equal?(x=w505, y=u16 5) -> (x >= y?=w508:bool)
        n339 = Not Equal?(x=w516, y=T8."待机") -> (x != y?=w515:bool)
        n340 = Select(t="", s=w515, f="加标模块启动加标\n判断加标是否启动成功" ("State(s) In (\"\")")) -> (s? t:f=w512:string)
        n341 = Select(t="流程结束" ("State(s) In (\"\")"), s=w508, f=w512) -> (s? t:f=w510:string)
        n342 = call "Add State to Queue.vi"("State(s) In Front (\"\")"=w510, "State(s) In (\"\")"=w519) -> ("States Out"=w518:string)  [unwired: 13 in]
      }
      frame "判断加标排液是否启动成功" {
        n343 = Index Array(array=w540, index=4 ("索引")) -> (element=w539:refnum<vi>)
        n344 = case shown="\"null\", 默认" w536 {
          tunnel: [T8."异常停机" ("运行状态") w554 w556 w558 w560 w562 w564 w566] -> w549
          frame "null", Default {
          }
          frame "氨氮" {
            n345 = global read "ZK非断电保存全局变量.vi" "氨氮质控仪器状态"() -> (w555:T12)
            n346 = Unbundle By Name(w555) -> ("运行状态"=w554:T8)
          }
          frame "总磷" {
            n347 = global read "ZK非断电保存全局变量.vi" "总磷质控仪器状态"() -> (w557:T12)
            n348 = Unbundle By Name(w557) -> ("运行状态"=w556:T8)
          }
          frame "总氮" {
            n349 = global read "ZK非断电保存全局变量.vi" "总氮质控仪器状态"() -> (w559:T12)
            n350 = Unbundle By Name(w559) -> ("运行状态"=w558:T8)
          }
          frame "CODMn" {
            n351 = global read "ZK非断电保存全局变量.vi" "CODMn质控仪器状态"() -> (w561:T12)
            n352 = Unbundle By Name(w561) -> ("运行状态"=w560:T8)
          }
          frame "CODCr" {
            n353 = global read "ZK非断电保存全局变量.vi" "CODCr质控仪器状态"() -> (w563:T12)
            n354 = Unbundle By Name(w563) -> ("运行状态"=w562:T8)
          }
          frame "氨氮总磷" {
            n355 = global read "ZK非断电保存全局变量.vi" "氨氮总磷质控仪器状态"() -> (w565:T12)
            n356 = Unbundle By Name(w565) -> ("运行状态"=w564:T8)
          }
          frame "总磷总氮" {
            n357 = global read "ZK非断电保存全局变量.vi" "总磷总氮质控仪器状态"() -> (w567:T12)
            n358 = Unbundle By Name(w567) -> ("运行状态"=w566:T8)
          }
        }
        n359 = property class="DigNum (严格)"(reference=w539) -> ("Value"=w538:u16)  [unwired: 1 in, 2 out]
        n360 = call "启动日志.vi"("日志信息"=w535, "Slave ID"=w536) -> ()  [unwired: 9 in, 1 out]
        n361 = Greater Or Equal?(x=w538, y=u16 5) -> (x >= y?=w541:bool)
        n362 = Not Equal?(x=w549, y=T8."待机") -> (x != y?=w548:bool)
        n363 = Select(t="", s=w548, f="加标模块启动排液\n判断加标是否启动成功" ("State(s) In (\"\")")) -> (s? t:f=w545:string)
        n364 = Select(t="流程结束" ("State(s) In (\"\")"), s=w541, f=w545) -> (s? t:f=w543:string)
        n365 = call "Add State to Queue.vi"("State(s) In Front (\"\")"=w543, "State(s) In (\"\")"=w552) -> ("States Out"=w551:string)  [unwired: 13 in]
      }
      frame "加标模块采样中", "加标模块加标中", "加标模块润洗中" {
        n366 = case shown="\"null\", 默认" w570 {
          tunnel: [T8."异常停机" ("运行状态") w585 w587 w589 w591 w593 w595 w597] -> w578
          frame "null", Default {
          }
          frame "氨氮" {
            n367 = global read "ZK非断电保存全局变量.vi" "氨氮质控仪器状态"() -> (w586:T12)
            n368 = Unbundle By Name(w586) -> ("运行状态"=w585:T8)
          }
          frame "总磷" {
            n369 = global read "ZK非断电保存全局变量.vi" "总磷质控仪器状态"() -> (w588:T12)
            n370 = Unbundle By Name(w588) -> ("运行状态"=w587:T8)
          }
          frame "总氮" {
            n371 = global read "ZK非断电保存全局变量.vi" "总氮质控仪器状态"() -> (w590:T12)
            n372 = Unbundle By Name(w590) -> ("运行状态"=w589:T8)
          }
          frame "CODMn" {
            n373 = global read "ZK非断电保存全局变量.vi" "CODMn质控仪器状态"() -> (w592:T12)
            n374 = Unbundle By Name(w592) -> ("运行状态"=w591:T8)
          }
          frame "CODCr" {
            n375 = global read "ZK非断电保存全局变量.vi" "CODCr质控仪器状态"() -> (w594:T12)
            n376 = Unbundle By Name(w594) -> ("运行状态"=w593:T8)
          }
          frame "氨氮总磷" {
            n377 = global read "ZK非断电保存全局变量.vi" "氨氮总磷质控仪器状态"() -> (w596:T12)
            n378 = Unbundle By Name(w596) -> ("运行状态"=w595:T8)
          }
          frame "总磷总氮" {
            n379 = global read "ZK非断电保存全局变量.vi" "总磷总氮质控仪器状态"() -> (w598:T12)
            n380 = Unbundle By Name(w598) -> ("运行状态"=w597:T8)
          }
        }
        n381 = First Call?() -> (First Call?: T/F=w568:bool)
        n382 = case shown="真" w568 {
          tunnel: w570 -> [_ w583]
          tunnel: w569 -> [_ w582]
          frame False {
          }
          frame True {
            n383 = call "启动日志.vi"("日志信息"=w582, "Slave ID"=w583) -> ()  [unwired: 9 in, 1 out]
          }
        }
        n384 = Equal?(x=w578, y=T8."等待取样") -> (x = y?=w576:bool)
        n385 = Select(t="", s=w576, f=w569) -> (s? t:f=w573:string)
        n386 = Equal?(x=w578, y=T8."异常停机") -> (x = y?=w574:bool)
        n387 = Select(t="流程结束" ("State(s) In (\"\")"), s=w574, f=w573) -> (s? t:f=w571:string)
        n388 = call "Add State to Queue.vi"("State(s) In Front (\"\")"=w571, "State(s) In (\"\")"=w581) -> ("States Out"=w580:string)  [unwired: 13 in]
      }
      frame "加标模块排液中" {
        n389 = case shown="\"null\", 默认" w601 {
          tunnel: [T8."异常停机" ("运行状态") w616 w618 w620 w622 w624 w626 w628] -> w609
          frame "null", Default {
          }
          frame "氨氮" {
            n390 = global read "ZK非断电保存全局变量.vi" "氨氮质控仪器状态"() -> (w617:T12)
            n391 = Unbundle By Name(w617) -> ("运行状态"=w616:T8)
          }
          frame "总磷" {
            n392 = global read "ZK非断电保存全局变量.vi" "总磷质控仪器状态"() -> (w619:T12)
            n393 = Unbundle By Name(w619) -> ("运行状态"=w618:T8)
          }
          frame "总氮" {
            n394 = global read "ZK非断电保存全局变量.vi" "总氮质控仪器状态"() -> (w621:T12)
            n395 = Unbundle By Name(w621) -> ("运行状态"=w620:T8)
          }
          frame "CODMn" {
            n396 = global read "ZK非断电保存全局变量.vi" "CODMn质控仪器状态"() -> (w623:T12)
            n397 = Unbundle By Name(w623) -> ("运行状态"=w622:T8)
          }
          frame "CODCr" {
            n398 = global read "ZK非断电保存全局变量.vi" "CODCr质控仪器状态"() -> (w625:T12)
            n399 = Unbundle By Name(w625) -> ("运行状态"=w624:T8)
          }
          frame "氨氮总磷" {
            n400 = global read "ZK非断电保存全局变量.vi" "氨氮总磷质控仪器状态"() -> (w627:T12)
            n401 = Unbundle By Name(w627) -> ("运行状态"=w626:T8)
          }
          frame "总磷总氮" {
            n402 = global read "ZK非断电保存全局变量.vi" "总磷总氮质控仪器状态"() -> (w629:T12)
            n403 = Unbundle By Name(w629) -> ("运行状态"=w628:T8)
          }
        }
        n404 = First Call?() -> (First Call?: T/F=w599:bool)
        n405 = case shown="真" w599 {
          tunnel: w601 -> [_ w614]
          tunnel: w600 -> [_ w613]
          frame False {
          }
          frame True {
            n406 = call "启动日志.vi"("日志信息"=w613, "Slave ID"=w614) -> ()  [unwired: 9 in, 1 out]
          }
        }
        n407 = Equal?(x=w609, y=T8."待机") -> (x = y?=w607:bool)
        n408 = Select(t="", s=w607, f=w600) -> (s? t:f=w604:string)
        n409 = Equal?(x=w609, y=T8."异常停机") -> (x = y?=w605:bool)
        n410 = Select(t="流程结束" ("State(s) In (\"\")"), s=w605, f=w604) -> (s? t:f=w602:string)
        n411 = call "Add State to Queue.vi"("State(s) In Front (\"\")"=w602, "State(s) In (\"\")"=w612) -> ("States Out"=w611:string)  [unwired: 13 in]
      }
      frame "-------------------# 仪器测试流程 #-------------------" {
        n412 = call "Add State to Queue.vi"("State(s) In (\"\")"=w631) -> ("States Out"=w630:string)  [unwired: 14 in]
      }
      frame "启动仪器水样测试" {
        n413 = case shown="\"总氮\"" w634 {
          frame "null", Default {
          }
          frame "氨氮" {
            n414 = call "氨氮启动器.vi"("控制命令"=enum16{"水样测试", "加标回收", "停止"}."水样测试") -> ()  [unwired: 11 in]
          }
          frame "总磷" {
            n415 = call "总磷启动器.vi"("控制命令"=enum16{"水样测试", "加标回收", "停止"}."水样测试") -> ()  [unwired: 11 in]
          }
          frame "总氮" {
            n416 = call "总氮启动器.vi"("控制命令"=enum16{"水样测试", "加标回收", "停止"}."水样测试") -> ()  [unwired: 11 in]
          }
          frame "CODMn" {
            n417 = call "CODmn启动器.vi"("控制命令"=enum16{"水样测试", "加标回收", "停止"}."水样测试") -> ()  [unwired: 11 in]
          }
        }
        n418 = Index Array(array=w637, index=5 ("索引")) -> (element=w636:refnum<vi>)
        n419 = property class="DigNum (严格)"(reference=w636) -> (reference out=w640:refnum<vi>, "Value"=w639:u16)  [unwired: 1 in, 1 out]
        n420 = Get Date/Time In Seconds() -> (seconds since 1Jan1904=→"水样测试启动时间":timestamp)
        n421 = call "启动日志.vi"("日志信息"=w633, "Slave ID"=w634) -> ()  [unwired: 9 in, 1 out]
        n422 = Increment(x=w639) -> (x+1=w638:u16)
        n423 = property class="DigNum (严格)"(reference=w640, "Value"=w638) -> ()  [unwired: 1 in, 2 out]
        n424 = call "Add State to Queue.vi"("State(s) In (\"\")"=w642) -> ("States Out"=w641:string)  [unwired: 14 in]
      }
      frame "启动仪器加标回收测试" {
        n425 = case shown="\"总磷\"" w649 {
          frame "null", Default {
          }
          frame "氨氮" {
            n426 = call "氨氮启动器.vi"("控制命令"=enum16{"水样测试", "加标回收", "停止"}."加标回收") -> ()  [unwired: 11 in]
          }
          frame "总磷" {
            n427 = call "总磷启动器.vi"("控制命令"=enum16{"水样测试", "加标回收", "停止"}."加标回收") -> ()  [unwired: 11 in]
          }
          frame "总氮" {
            n428 = call "总氮启动器.vi"("控制命令"=enum16{"水样测试", "加标回收", "停止"}."加标回收") -> ()  [unwired: 11 in]
          }
          frame "CODMn" {
            n429 = call "CODmn启动器.vi"("控制命令"=enum16{"水样测试", "加标回收", "停止"}."加标回收") -> ()  [unwired: 11 in]
          }
        }
        n430 = Index Array(array=w652, index=6 ("索引")) -> (element=w651:refnum<vi>)
        n431 = property class="DigNum (严格)"(reference=w651) -> (reference out=w655:refnum<vi>, "Value"=w654:u16)  [unwired: 1 in, 1 out]
        n432 = call "启动日志.vi"("日志信息"=w648, "Slave ID"=w649) -> ()  [unwired: 9 in, 1 out]
        n433 = Get Date/Time In Seconds() -> (seconds since 1Jan1904=→"加标回收启动时间":timestamp)
        n434 = Increment(x=w654) -> (x+1=w653:u16)
        n435 = property class="DigNum (严格)"(reference=w655, "Value"=w653) -> ()  [unwired: 1 in, 2 out]
        n436 = call "Add State to Queue.vi"("State(s) In (\"\")"=w657) -> ("States Out"=w656:string)  [unwired: 14 in]
      }
      frame "exit" {
        n437 = flat-sequence {
          tunnel: w662 -> [w667]
          frame #0 {
            n438 = global read "ZK非断电保存全局变量.vi" "流程运行状态标记位"() -> (w668:T4)
            n439 = case shown="\"氨氮\"" w667 {
              tunnel: w668 -> [_ w671 w672 w675 w678 w681]
              frame "null", Default {
              }
              frame "氨氮" {
                n440 = Bundle By Name(cluster=w671, "氨氮"=FALSE) -> (w670:T4)
                n441 = global write "ZK非断电保存全局变量.vi" "流程运行状态标记位"(w670) -> ()
              }
              frame "总磷" {
                n442 = Bundle By Name(cluster=w672, "总磷"=FALSE ("氨氮")) -> (w674:T4)
                n443 = global write "ZK非断电保存全局变量.vi" "流程运行状态标记位"(w674) -> ()
              }
              frame "总氮" {
                n444 = Bundle By Name(cluster=w675, "总氮"=FALSE ("氨氮")) -> (w677:T4)
                n445 = global write "ZK非断电保存全局变量.vi" "流程运行状态标记位"(w677) -> ()
              }
              frame "CODMn" {
                n446 = Bundle By Name(cluster=w678, "CODMn"=FALSE ("氨氮")) -> (w680:T4)
                n447 = global write "ZK非断电保存全局变量.vi" "流程运行状态标记位"(w680) -> ()
              }
              frame "CODCr" {
                n448 = Bundle By Name(cluster=w681, "CODCr"=FALSE ("氨氮")) -> (w683:T4)
                n449 = global write "ZK非断电保存全局变量.vi" "流程运行状态标记位"(w683) -> ()
              }
            }
          }
          frame #1 {
            n450 = global read "ZK非断电保存全局变量.vi" "流程运行状态标记位"() -> (w687:T4)
            n451 = Cluster To Array(cluster=w687) -> (array=w686:bool[])
            n452 = Boolean Array To Number(Boolean array=w686) -> (number=w685:u32)
            n453 = Equal To 0?(x=w685) -> (x = 0?=w684:bool)
            n454 = case shown="真" w684 {
              frame False {
              }
              frame True {
                n455 = call "采配水启动器.vi"("启动/停止命令"=enum16{"待机", "水样测试", "停止", "加标回收"}."停止") -> ()  [unwired: 10 in, 1 out]
              }
            }
          }
        }
        n456 = case shown="\"null\", 默认" w662 {
          frame "null", Default {
          }
          frame "氨氮" {
            n457 = call "氨氮启动器.vi"("控制命令"=enum16{"水样测试", "加标回收", "停止"}."停止") -> ()  [unwired: 11 in]
          }
          frame "总磷" {
            n458 = call "总磷启动器.vi"("控制命令"=enum16{"水样测试", "加标回收", "停止"}."停止") -> ()  [unwired: 11 in]
          }
          frame "总氮" {
            n459 = call "总氮启动器.vi"("控制命令"=enum16{"水样测试", "加标回收", "停止"}."停止") -> ()  [unwired: 11 in]
          }
          frame "CODMn" {
            n460 = call "CODmn启动器.vi"("控制命令"=enum16{"水样测试", "加标回收", "停止"}."停止") -> ()  [unwired: 11 in]
          }
        }
        n461 = call "启动日志.vi"("日志信息"=w664, "Slave ID"=w662) -> ()  [unwired: 9 in, 1 out]
        n462 = call "Add State to Queue.vi"("State(s) In Front (\"\")"="流程结束" ("State(s) In Front (\"\")"), "State(s) In (\"\")"=w666) -> ("States Out"=w665:string)  [unwired: 13 in]
      }
      frame "判断仪器水样是否启动成功" {
        n463 = case shown="\"氨氮\"" w694 {
          tunnel: [T9."空闲" ("工作状态") w713 w715 w717 w719] -> w708
          frame "null", Default {
          }
          frame "氨氮" {
            w712 = u16 3 items=["总磷"=1, "总氮"=2, "氨氮"=3, "CODMn"=21] ("站号")
            n464 = call "获取仪器仪表状态.vi"("站号"=w712) -> ("工作状态"=w713:T9)  [unwired: 10 in]
          }
          frame "总磷" {
            w714 = u16 1 items=["总磷"=1, "总氮"=2, "氨氮"=3, "CODMn"=21] ("站号")
            n465 = call "获取仪器仪表状态.vi"("站号"=w714) -> ("工作状态"=w715:T9)  [unwired: 10 in]
          }
          frame "总氮" {
            w716 = u16 2 items=["总磷"=1, "总氮"=2, "氨氮"=3, "CODMn"=21] ("站号")
            n466 = call "获取仪器仪表状态.vi"("站号"=w716) -> ("工作状态"=w717:T9)  [unwired: 10 in]
          }
          frame "CODMn" {
            w718 = u16 21 items=["总磷"=1, "总氮"=2, "氨氮"=3, "CODMn"=21] ("站号")
            n467 = call "获取仪器仪表状态.vi"("站号"=w718) -> ("工作状态"=w719:T9)  [unwired: 10 in]
          }
        }
        n468 = Index Array(array=w698, index=5 ("索引")) -> (element=w697:refnum<vi>)
        n469 = call "启动日志.vi"("日志信息"=w693, "Slave ID"=w694) -> ()  [unwired: 9 in, 1 out]
        n470 = property class="DigNum (严格)"(reference=w697) -> ("Value"=w696:u16)  [unwired: 1 in, 2 out]
        n471 = Greater Or Equal?(x=w696, y=u16 5) -> (x >= y?=w702:bool)
        n472 = Equal?(x=w708, y=T9."空闲") -> (x = y?=w706:bool)
        n473 = Select(t="启动仪器水样测试\n判断仪器水样是否启动成功" ("State(s) In (\"\")"), s=w706, f="") -> (s? t:f=w700:string)
        n474 = Select(t="流程结束" ("State(s) In (\"\")"), s=w702, f=w700) -> (s? t:f=w699:string)
        n475 = call "Add State to Queue.vi"("State(s) In Front (\"\")"=w699, "State(s) In (\"\")"=w710) -> ("States Out"=w709:string)  [unwired: 13 in]
      }
      frame "判断仪器加标是否启动成功" {
        n476 = case shown="\"氨氮\"" w721 {
          tunnel: [T9."空闲" ("工作状态") w740 w742 w744 w746] -> w722
          frame "null", Default {
          }
          frame "氨氮" {
            w739 = u16 3 items=["总磷"=1, "总氮"=2, "氨氮"=3, "CODMn"=21] ("站号")
            n477 = call "获取仪器仪表状态.vi"("站号"=w739) -> ("工作状态"=w740:T9)  [unwired: 10 in]
          }
          frame "总磷" {
            w741 = u16 1 items=["总磷"=1, "总氮"=2, "氨氮"=3, "CODMn"=21] ("站号")
            n478 = call "获取仪器仪表状态.vi"("站号"=w741) -> ("工作状态"=w742:T9)  [unwired: 10 in]
          }
          frame "总氮" {
            w743 = u16 2 items=["总磷"=1, "总氮"=2, "氨氮"=3, "CODMn"=21] ("站号")
            n479 = call "获取仪器仪表状态.vi"("站号"=w743) -> ("工作状态"=w744:T9)  [unwired: 10 in]
          }
          frame "CODMn" {
            w745 = u16 21 items=["总磷"=1, "总氮"=2, "氨氮"=3, "CODMn"=21] ("站号")
            n480 = call "获取仪器仪表状态.vi"("站号"=w745) -> ("工作状态"=w746:T9)  [unwired: 10 in]
          }
        }
        n481 = Index Array(array=w726, index=6 ("索引")) -> (element=w725:refnum<vi>)
        n482 = call "启动日志.vi"("日志信息"=w720, "Slave ID"=w721) -> ()  [unwired: 9 in, 1 out]
        n483 = property class="DigNum (严格)"(reference=w725) -> ("Value"=w724:u16)  [unwired: 1 in, 2 out]
        n484 = Greater Or Equal?(x=w724, y=u16 5) -> (x >= y?=w729:bool)
        n485 = Equal?(x=w722, y=T9."空闲") -> (x = y?=w734:bool)
        n486 = Select(t="启动仪器加标回收测试\n判断仪器加标是否启动成功" ("State(s) In (\"\")"), s=w734, f="") -> (s? t:f=w728:string)
        n487 = Select(t="流程结束" ("State(s) In (\"\")"), s=w729, f=w728) -> (s? t:f=w727:string)
        n488 = call "Add State to Queue.vi"("State(s) In Front (\"\")"=w727, "State(s) In (\"\")"=w737) -> ("States Out"=w736:string)  [unwired: 13 in]
      }
      frame "仪器加标回收测试中", "仪器水样测试中" {
        n489 = case shown="\"氨氮\"" w748 {
          tunnel: [T9."空闲" ("工作状态") w759 w761 w763 w765] -> w747
          frame "null", Default {
          }
          frame "氨氮" {
            w758 = u16 3 items=["总磷"=1, "总氮"=2, "氨氮"=3, "CODMn"=21] ("站号")
            n490 = call "获取仪器仪表状态.vi"("站号"=w758) -> ("工作状态"=w759:T9)  [unwired: 10 in]
          }
          frame "总磷" {
            w760 = u16 1 items=["总磷"=1, "总氮"=2, "氨氮"=3, "CODMn"=21] ("站号")
            n491 = call "获取仪器仪表状态.vi"("站号"=w760) -> ("工作状态"=w761:T9)  [unwired: 10 in]
          }
          frame "总氮" {
            w762 = u16 2 items=["总磷"=1, "总氮"=2, "氨氮"=3, "CODMn"=21] ("站号")
            n492 = call "获取仪器仪表状态.vi"("站号"=w762) -> ("工作状态"=w763:T9)  [unwired: 10 in]
          }
          frame "CODMn" {
            w764 = u16 21 items=["总磷"=1, "总氮"=2, "氨氮"=3, "CODMn"=21] ("站号")
            n493 = call "获取仪器仪表状态.vi"("站号"=w764) -> ("工作状态"=w765:T9)  [unwired: 10 in]
          }
        }
        n494 = First Call?() -> (First Call?: T/F=w749:bool)
        n495 = case shown="真" w749 {
          tunnel: w748 -> [_ w767]
          tunnel: w750 -> [_ w766]
          frame False {
          }
          frame True {
            n496 = call "启动日志.vi"("日志信息"=w766, "Slave ID"=w767) -> ()  [unwired: 9 in, 1 out]
          }
        }
        n497 = Equal?(x=w747, y=T9."空闲") -> (x = y?=w753:bool)
        n498 = Select(t="", s=w753, f=w750) -> (s? t:f=w751:string)
        n499 = call "Add State to Queue.vi"("State(s) In Front (\"\")"=w751, "State(s) In (\"\")"=w756) -> ("States Out"=w755:string)  [unwired: 13 in]
      }
    }
  }
